vi "Initialize Coerce.vi"(8 "error in (no error)":errorcluster, 11 "Numeric Data Type in":refnum<class "Numeric Data Type.lvclass">) -> (0 "error out":errorcluster, 3 "Numeric Data Type (dup)":refnum<class "Numeric Data Type.lvclass">)   [LabVIEW 2018, in "Numeric Data Type.lvclass"]
uses:
  Numeric Data Type.lvclass
  Numeric Data Type.lvclass/Numeric Data Type.ctl
  Reference Coerce Increment.vi
  Reference Coerce Maximum.vi
  Reference Coerce Minimum.vi
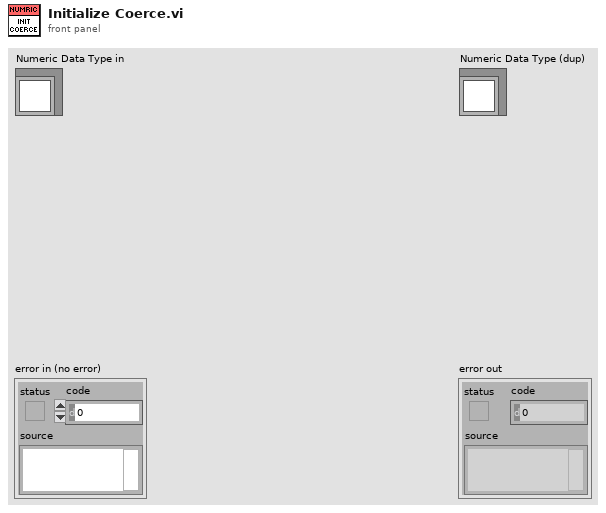
[diagram p1: front panel]
types:
  T1 = typedef "Numeric Data Type.lvclass/Representation Enum.ctl" = enum16{"Extended (EXT)", "Double (DBL)", "Single (SGL)", "Fixed-Point (FXP)", "Quad Integer (I64)", "Long Integer (I32)", "Word Integer (I16)", "Byte Integer (I8)", "Unsigned Quad (U64)", "Unsigned Long (U32)", "Unsigned Word (U16)", "Unsigned Byte (U8)", "Complex Extended (CXT)", "Complex Double (CDB)", "Complex Single (CSG)"}
  T2 = typedef "Numeric Data Type.lvclass/Response to Values Outside of Limits Enum.ctl" = enum16{"Ignore", "Coerce to nearest", "Coerce up", "Coerce down"}
  T3 = enum8{"Enabled", "Disabled", "Disabled and Grayed Out"}
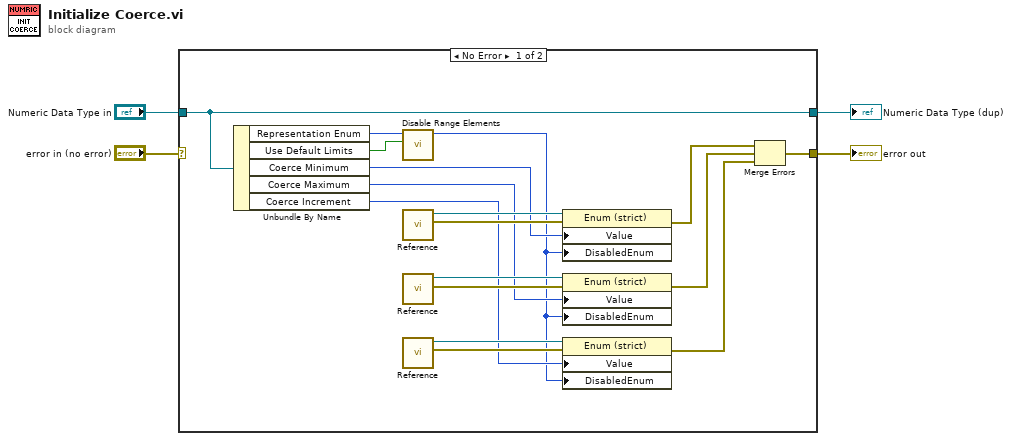
[diagram p0: block diagram]
diagram:
  n1 = case shown="No Error" "error in (no error)" {
    selector: "error in (no error)" -> [_ w23]
    tunnel: [w9 w23] -> w3
    tunnel: [w15 w22] -> w1
    tunnel: "Numeric Data Type in" -> [w15 w22]
    frame No Error {
      n2 = Unbundle By Name(w15) -> ("Representation Enum"=w14:T1, "Use Default Limits"=w13:bool, "Coerce Minimum"=w12:T2, "Coerce Maximum"=w11:T2, "Coerce Increment"=w10:T2)
      n3 = call "Disable Range Elements.vi"("Use Default Limits"=w13, "Representation Enum"=w14) -> ("Disabled?"=w5:T3)  [unwired: 9 in]
      n4 = call-poly "Reference.vi"() -> ("error out"=w19:errorcluster, "Coerce Minimum"=w16:refnum<vi>)  [unwired: 10 in]
      n5 = call-poly "Reference.vi"() -> ("error out"=w18:errorcluster, "Coerce Maximum"=w17:refnum<vi>)  [unwired: 10 in]
      n6 = call-poly "Reference.vi"() -> ("error out"=w21:errorcluster, "Coerce Increment"=w20:refnum<vi>)  [unwired: 10 in]
      n7 = property class="Enum (strict)"(reference=w16, error in=w19, "Value"=w12, "DisabledEnum"=w5) -> (error out=w8:errorcluster)  [unwired: 1 out]
      n8 = property class="Enum (strict)"(reference=w17, error in=w18, "Value"=w11, "DisabledEnum"=w5) -> (error out=w7:errorcluster)  [unwired: 1 out]
      n9 = property class="Enum (strict)"(reference=w20, error in=w21, "Value"=w10, "DisabledEnum"=w5) -> (error out=w6:errorcluster)  [unwired: 1 out]
      n10 = Merge Errors(w8, w7, w6) -> (w9:errorcluster)
    }
    frame Error {
    }
  }
  "error out" <- w3
  "Numeric Data Type (dup)" <- w1
